vi "GetDeviceParameterInfo.vi"(8 "error in":errorcluster, 9 "Parameter Name":string, 10 "Device Command":string, 11 "connection ID in":refnum<k5>) -> (0 "error out":errorcluster, 1 "Error Info":T1, 2 "Device Parameter Info":T2, 3 "connection ID out":refnum<k5>, 4 "Log String":string, 5 "OK":bool)   [LabVIEW 2015, in "ProdigyRemoteControl.lvlib"]
uses:
  ProdigyRemoteControl.lvlib
  DEFINITIONS/DEF_DeviceParaInfo.ctl
  DEFINITIONS/DEF_RcError.ctl
  DEFINITIONS/DEF_RcCmd.ctl
  <vilib>/regexp/Match Regular Expression.xnode
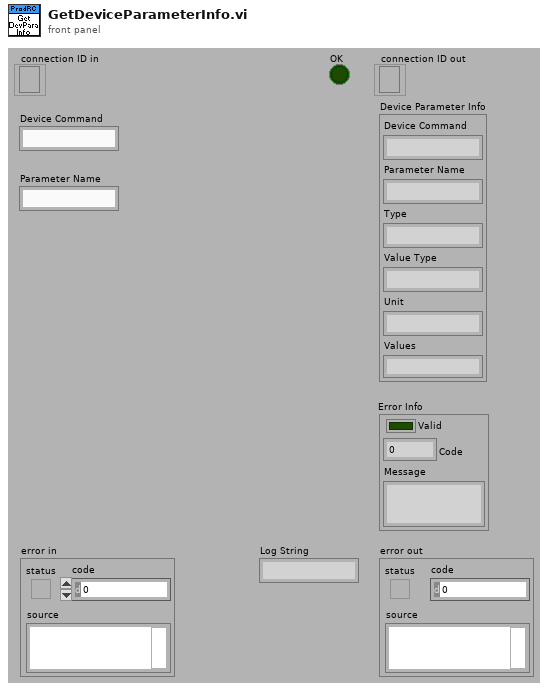
[diagram p1: front panel]
types:
  T1 = typedef "ProdigyRemoteControl.lvlib/DEF_RcError.ctl" = cluster{"Valid":bool, "Code":u16, "Message":string}
  T2 = typedef "ProdigyRemoteControl.lvlib/DEF_DeviceParaInfo.ctl" = cluster{"Device Command":string, "Parameter Name":string, "Type":string, "Value Type":string, "Unit":string, "Values":string}
  T3 = typedef "ProdigyRemoteControl.lvlib/DEF_RcCmd.ctl" = string
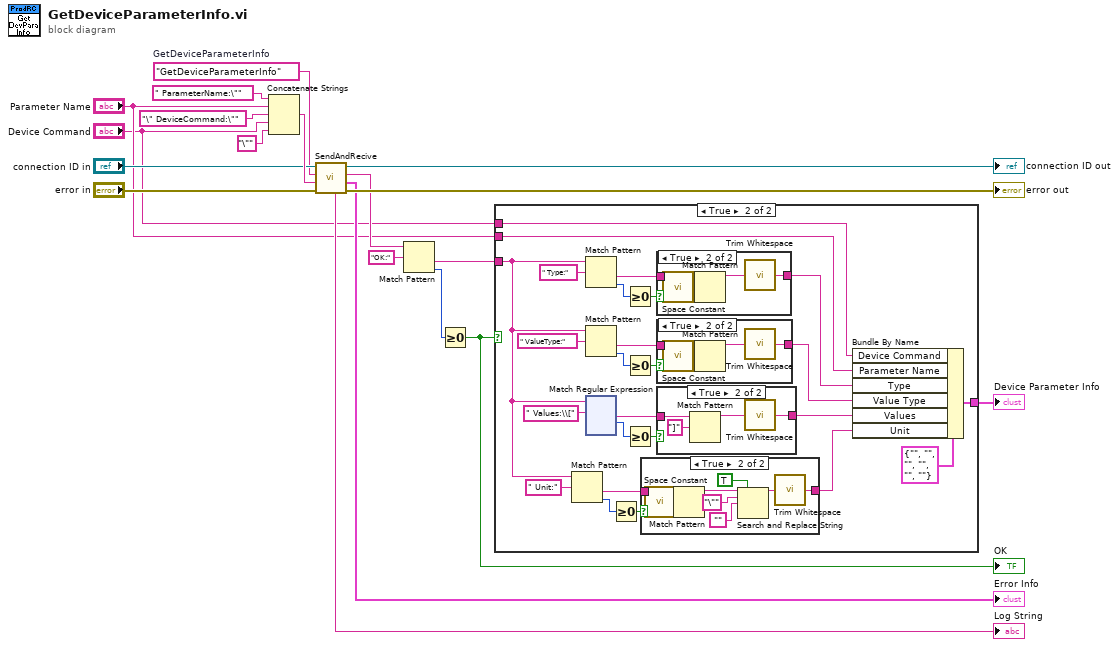
[diagram p0: block diagram]
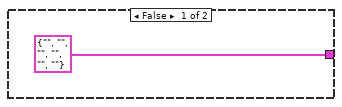
[diagram p2: hidden frame]
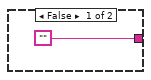
[diagram p3: hidden frame]
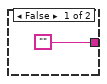
[diagram p4: hidden frame]
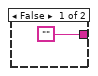
[diagram p5: hidden frame]
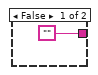
[diagram p6: hidden frame]
diagram:
  w4 = T3 "GetDeviceParameterInfo"  # GetDeviceParameterInfo
  n1 = Concatenate Strings(" ParameterName:\"", "Parameter Name", "\" DeviceCommand:\"" ("string"), "Device Command", "\"" ("string")) -> (w19:string)
  n2 = call "SendAndRecive.vi"("error in"="error in", "Parameters"=w19, "Command"=w4, "connection ID in"="connection ID in") -> ("error out"=→"error out":errorcluster, "Error Info"=→"Error Info":T1, "Answer"=w11:string, "connection ID out"=→"connection ID out":refnum<k5>, "Log String"=→"Log String":string)  [unwired: 3 in]
  n3 = Match Pattern(string=w11, regular expression="OK:") -> (after substring=w7:string, offset past match=w9:i32)  [unwired: 1 in, 2 out]
  n4 = Greater Or Equal To 0?(x=w9) -> (x >= 0?=w8:bool)
  "OK" <- w8
  n5 = case shown="True" w8 {
    tunnel: w7 -> [_ w25]
    tunnel: "Parameter Name" -> [_ w31]
    tunnel: [T2 {"Device Command"="", "Parameter Name"="", "Type"="", "Value Type"="", "Unit"="", "Values"=""} ("DEF_ParameterInfo") w28] -> w5
    tunnel: "Device Command" -> [_ w22]
    frame False {
    }
    frame True {
      n6 = Match Pattern(string=w25, regular expression=" Unit:") -> (after substring=w36:string, offset past match=w37:i32)  [unwired: 1 in, 2 out]
      n7 = Match Pattern(string=w25, regular expression=" Type:") -> (after substring=w42:string, offset past match=w44:i32)  [unwired: 1 in, 2 out]
      n8 = Match Pattern(string=w25, regular expression=" ValueType:") -> (after substring=w39:string, offset past match=w38:i32)  [unwired: 1 in, 2 out]
      n9 = xnode "Match Regular Expression"("input string"=w25, "regular expression"=" Values:\\[") -> ("after match"=w24:string, "offset past match"=w23:i32)  [unwired: 4 in, 3 out]
      n10 = Greater Or Equal To 0?(x=w37) -> (x >= 0?=w34:bool)
      n11 = Greater Or Equal To 0?(x=w44) -> (x >= 0?=w43:bool)
      n12 = Greater Or Equal To 0?(x=w38) -> (x >= 0?=w41:bool)
      n13 = Greater Or Equal To 0?(x=w23) -> (x >= 0?=w33:bool)
      n14 = case shown="True" w34 {
        tunnel: w36 -> [_ w170]
        tunnel: ["" w163] -> w27
        frame False {
        }
        frame True {
          n15 = call <vilib>:"Space Constant.vi"() -> ("String"=w169:string)
          n16 = Match Pattern(string=w170, regular expression=w169) -> (before substring=w167:string)  [unwired: 1 in, 3 out]
          n17 = Search and Replace String(replace all?=TRUE ("replace all? (F)"), input string=w167, search string="\"", replace string="") -> (result string=w168:string)  [unwired: 4 in, 3 out]
          n18 = call <vilib>:"Trim Whitespace.vi"("string"=w168) -> ("trimmed string"=w163:string)  [unwired: 1 in]
        }
      }
      n19 = case shown="True" w43 {
        tunnel: w42 -> [_ w180]
        tunnel: ["" w178] -> w30
        frame False {
        }
        frame True {
          n20 = call <vilib>:"Space Constant.vi"() -> ("String"=w179:string)
          n21 = Match Pattern(string=w180, regular expression=w179) -> (before substring=w177:string)  [unwired: 1 in, 3 out]
          n22 = call <vilib>:"Trim Whitespace.vi"("string"=w177) -> ("trimmed string"=w178:string)  [unwired: 1 in]
        }
      }
      n23 = case shown="True" w41 {
        tunnel: w39 -> [_ w175]
        tunnel: ["" w173] -> w29
        frame False {
        }
        frame True {
          n24 = call <vilib>:"Space Constant.vi"() -> ("String"=w174:string)
          n25 = Match Pattern(string=w175, regular expression=w174) -> (before substring=w172:string)  [unwired: 1 in, 3 out]
          n26 = call <vilib>:"Trim Whitespace.vi"("string"=w172) -> ("trimmed string"=w173:string)  [unwired: 1 in]
        }
      }
      n27 = case shown="True" w33 {
        tunnel: w24 -> [_ w161]
        tunnel: ["" w159] -> w21
        frame False {
        }
        frame True {
          n28 = Match Pattern(string=w161, regular expression="]") -> (before substring=w158:string)  [unwired: 1 in, 3 out]
          n29 = call <vilib>:"Trim Whitespace.vi"("string"=w158) -> ("trimmed string"=w159:string)  [unwired: 1 in]
        }
      }
      n30 = Bundle By Name(cluster=T2 {"Device Command"="", "Parameter Name"="", "Type"="", "Value Type"="", "Unit"="", "Values"=""} ("DEF_ParameterInfo"), "Device Command"=w22, "Parameter Name"=w31, "Type"=w30, "Value Type"=w29, "Values"=w21, "Unit"=w27) -> (w28:T2)
    }
  }
  "Device Parameter Info" <- w5
